vi "Convert RAWDATA.vi"(0 "Detector in":refnum<class "Detector.lvclass">, 1 "I channel":sgl[][](array[numeric]), 3 "WCM_values IN":sgl[](array[numeric]), 4 "II channel":sgl[][](array[numeric]), 5 "error in (no error)":errorcluster, 6 "# of scan":i32, 7 "All?":bool=TRUE, 10 "WCM_limits":T1, 11 "WCM_corrections":bool, 12 "I channel seq IN":cluster{"BG":sgl[], "Ie":sgl[], "I0":sgl[]}[](array[cluster]), 13 "II channel seq IN":cluster{"BG":sgl[], "Ie":sgl[], "I0":sgl[]}[](array[cluster])) -> (14 "Detector out":refnum<class "Detector.lvclass">, 15 "I channel seq":cluster{"BG":sgl[], "Ie":sgl[], "I0":sgl[]}[](array[cluster]), 17 "WCM_correction_coff":sgl[](array[numeric]), 18 "II channel seq":cluster{"BG":sgl[], "Ie":sgl[], "I0":sgl[]}[](array[cluster]), 19 "error out":errorcluster)   [LabVIEW 2020, in "Detector.lvclass"]
uses:
  Detector.lvclass
  dependecies/ControlsVIs/Clusters-def/Def_WCM_limits.ctl
  Detector.lvclass/Detector.ctl
  Read SC sum values ref.vi
  dependecies/globalVarII.vi
  <userlib>/_OpenG.lib/array/array.llb/Search 1D Array (SGL)__ogtk.vi
  Oscilloscope/Oscilloscope.lvclass
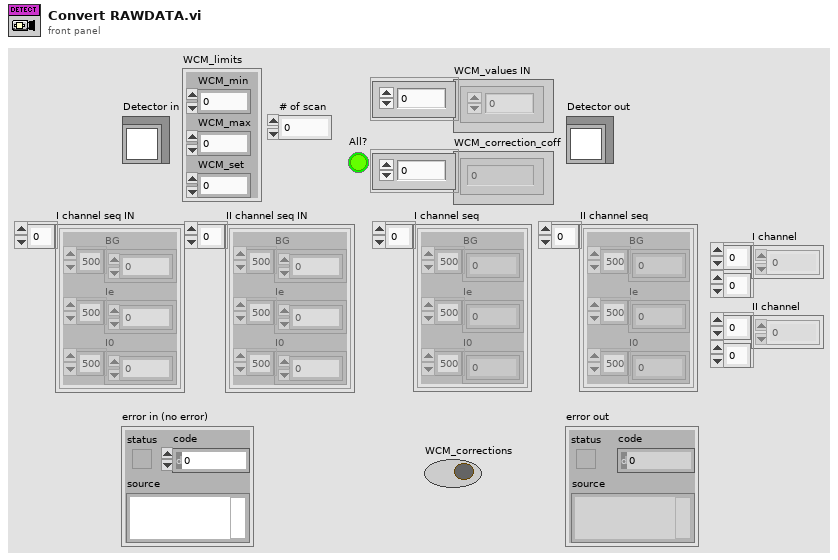
[diagram p1: front panel]
types:
  T1 = typedef "Oscilloscope.lvclass/Def_WCM_limits.ctl" = cluster{"WCM_min":dbl, "WCM_max":dbl, "WCM_set":dbl}
  T2 = typedef "Control-Client.lvclass/Controls-refs_CLIENT.ctl" = cluster{"ON/OFF Cool":refnum<vi>, "Save spectra":refnum<vi>, "Read detector":refnum<vi>, "# scans":refnum<vi>, "BG-level":refnum<vi>, "Set T":refnum<vi>, "Termometer":refnum<vi>, "Spectra":refnum<vi>, "Error Meter_ref":refnum<vi>, "OD graph":refnum<vi>, "from_pixel":refnum<vi>, "to_pixel":refnum<vi>, "threshold_ref_channel":refnum<vi>, "value":refnum<vi>, "python session":refnum<vi>, "ref h5_file":T3, "distance":refnum<vi>}
  T3 = typedef "hid_t.ctl" = i64
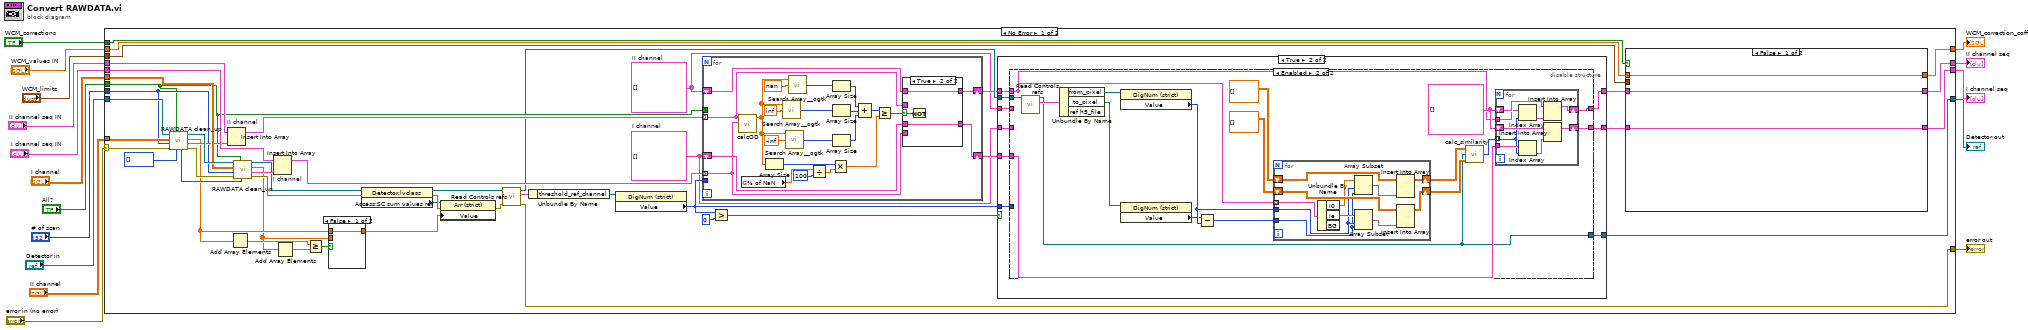
[diagram p0: block diagram]
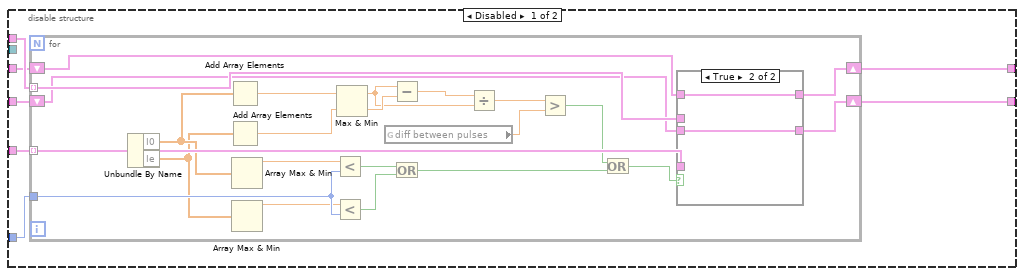
[diagram p3: hidden frame]
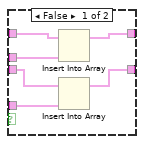
[diagram p4: hidden frame]
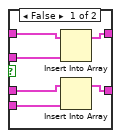
[diagram p5: hidden frame]
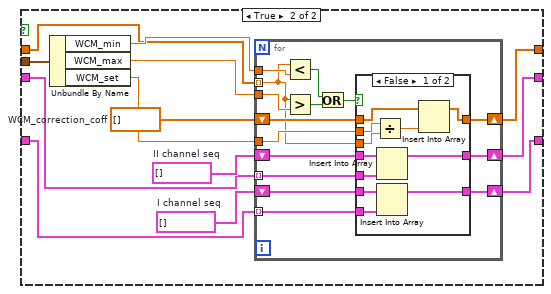
[diagram p7: hidden frame]
diagram:
  n1 = case shown="No Error" "error in (no error)" {
    selector: "error in (no error)" -> [w56 w235]
    tunnel: [w17 w236] -> w13
    tunnel: "Detector in" -> [w55 w236]
    tunnel: [w18 w235] -> w12
    tunnel: [w64 w234] -> w16
    tunnel: [w63 w233] -> w15
    tunnel: "II channel seq IN" -> [w62 w234]
    tunnel: "I channel seq IN" -> [w61 w233]
    tunnel: [w60 w232] -> w5
    tunnel: "WCM_values IN" -> [w59 w232]
    tunnel: "I channel" -> [w45 _]
    tunnel: "II channel" -> [w47 _]
    tunnel: "WCM_corrections" -> [w58 _]
    tunnel: "WCM_limits" -> [w57 _]
    tunnel: "All?" -> [w31 _]
    tunnel: "# of scan" -> [w38 _]
    frame No Error {
      w21 = cluster{"BG":sgl[], "Ie":sgl[], "I0":sgl[]}[] []  # II channel
      w22 = cluster{"BG":sgl[], "Ie":sgl[], "I0":sgl[]}[] []  # I channel
      n2 = call "RAWDATA clean_up.vi"("BG index IN"=i32[] [], "All?"=w31, "error in (no error)"=w56, "# of scan"=w38, "channel"=w47, "Detector in"=w55) -> ("error out"=w49:errorcluster, "channel seq"=w43:cluster{"BG":i32[], "Ie":i32[], "I0":i32[]}[], "SC values"=w39:sgl[], "Detector out"=w48:refnum<class "Detector.lvclass">, "BG indexes"=w46:i32[])  [unwired: 1 in]
      n3 = Insert Into Array "II channel"(array=w62, new element=w43) -> (w35:cluster{"BG":sgl[], "Ie":sgl[], "I0":sgl[]}[])  [unwired: 1 in]
      n4 = Add Array Elements(numeric array=w39) -> (sum=w52:sgl)
      n5 = call "RAWDATA clean_up.vi"("BG index IN"=w46, "All?"=w31, "error in (no error)"=w49, "# of scan"=w38, "channel"=w45, "Detector in"=w48) -> ("error out"=w41:errorcluster, "channel seq"=w44:cluster{"BG":i32[], "Ie":i32[], "I0":i32[]}[], "SC values"=w32:sgl[], "Detector out"=w42:refnum<class "Detector.lvclass">)  [unwired: 1 in, 1 out]
      n6 = Insert Into Array "I channel"(array=w61, new element=w44) -> (w36:cluster{"BG":sgl[], "Ie":sgl[], "I0":sgl[]}[])  [unwired: 1 in]
      n7 = Add Array Elements(numeric array=w32) -> (sum=w51:sgl)
      n8 = Greater Or Equal?(x=w52, y=w51) -> (x >= y?=w50:bool)
      n9 = case shown="False" w50 {
        tunnel: w39 -> [w185 _]
        tunnel: [w185 w186] -> w40
        tunnel: w32 -> [_ w186]
        frame False {
        }
        frame True {
        }
      }
      n10 = property class="Detector.lvclass"(reference=w42, error in=w41) -> (reference out=w29:refnum<class "Detector.lvclass">, error out=w54:errorcluster, "Access:SC sum values ref"=w53:refnum<vi>)
      n11 = property class="Arr (strict)"(reference=w53, error in=w54, "Value"=w40) -> (error out=w30:errorcluster)  [unwired: 1 out]
      n12 = call "Read Controls refs.vi"("error in (no error)"=w30, "Detector in"=w29) -> ("error out"=w18:errorcluster, "Controls refs"=w28:T2, "Detector out"=w25:refnum<class "Detector.lvclass">)  [unwired: 7 in]
      n13 = Unbundle By Name(w28) -> ("threshold_ref_channel"=w27:refnum<vi>)
      n14 = property class="DigNum (strict)"(reference=w27) -> ("Value"=w26:i32)  [unwired: 1 in, 2 out]
      n15 = for {
        tunnel: w36 -> [w155] mode=indexing
        tunnel: w35 -> [w165] mode=indexing
        shift-right: [w153] -> w23
        shift-left: w22 -> [w167]
        shift-right: [w154] -> w24
        shift-left: w21 -> [w166]
        tunnel: w31 -> [_]
        tunnel: w26 -> [_]
        n16 = call "calcOD.vi"("channel I"=w155, "channel 2"=w165) -> ("OD"=w173:sgl[])  [unwired: 3 in, 6 out]
        n17 = global read "globalVarII.vi" "% of NaN"() -> (w163:sgl)
        n18 = Array Size(array=w173) -> (size(s)=w172:i32)
        n19 = call-poly <userlib>:"Search Array__ogtk.vi"("Array"=w173, "Element Data"=sgl inf) -> ("Indices of Elements"=w171:i32[])  [unwired: 7 in]
        n20 = call-poly <userlib>:"Search Array__ogtk.vi"("Array"=w173, "Element Data"=sgl -inf) -> ("Indices of Elements"=w170:i32[])  [unwired: 7 in]
        n21 = call-poly <userlib>:"Search Array__ogtk.vi"("Array"=w173, "Element Data"=sgl nan) -> ("Indices of Elements"=w174:i32[])  [unwired: 7 in]
        n22 = Divide(x=w163, y=100) -> (x/y=w164:sgl)
        n23 = Multiply(x=w172, y=w164) -> (x*y=w157:sgl)
        n24 = Array Size(array=w174) -> (size(s)=w161:i32)
        n25 = Array Size(array=w171) -> (size(s)=w160:i32)
        n26 = Array Size(array=w170) -> (size(s)=w159:i32)
        n27 = Compound Arithmetic op=ADD(w161, w160, w159) -> (w158:i32)
        n28 = Greater Or Equal?(x=w158, y=w157) -> (x >= y?=w156:bool)
        n29 = case shown="True" w156 {
          selector: w156 -> [_ w182]
          tunnel: w167 -> [w181 w183]
          tunnel: w155 -> [w180 _]
          tunnel: [w179 w183] -> w153
          tunnel: [w178 w184] -> w154
          tunnel: w166 -> [w177 w184]
          tunnel: w165 -> [w176 _]
          frame False {
            n30 = Insert Into Array(array=w177, new element=w176) -> (w178:cluster{"BG":sgl[], "Ie":sgl[], "I0":sgl[]}[])  [unwired: 1 in]
            n31 = Insert Into Array(array=w181, new element=w180) -> (w179:cluster{"BG":sgl[], "Ie":sgl[], "I0":sgl[]}[])  [unwired: 1 in]
          }
          frame True {
            n32 = Not(x=w182) -> ()  [unwired: 1 out]
          }
        }
      }
      n33 = Greater?(x=w26, y=0) -> (0:w19:bool)
      n34 = case shown="True" w19 {
        tunnel: [w67 w72] -> w33
        tunnel: w24 -> [w67 w76]
        tunnel: w23 -> [w66 w75]
        tunnel: [w66 w71] -> w34
        tunnel: w22 -> [_ w74]
        tunnel: w21 -> [_ w73]
        tunnel: w26 -> [_ w70]
        tunnel: w25 -> [w65 w69]
        tunnel: [w65 w68] -> w17
        frame False {
        }
        frame True {
          n35 = disable-structure shown="Enabled" {
            disable-tunnel: w76 -> [w83 w126]
            disable-tunnel: w75 -> [w82 w129]
            disable-tunnel: w74 -> [w81 _]
            disable-tunnel: w73 -> [w80 _]
            disable-tunnel: [w79 w125] -> w72
            disable-tunnel: [w78 w128] -> w71
            disable-tunnel: w70 -> [w77 _]
            disable-tunnel: w69 -> [_ w121]
            disable-tunnel: [_ w115] -> w68
            frame Disabled {
              n36 = for {
                tunnel: w83 -> [w102] mode=indexing
                tunnel: w82 -> [w101] mode=indexing
                shift-right: [w99] -> w78
                shift-left: w81 -> [w100]
                shift-right: [w103] -> w79
                shift-left: w80 -> [w104]
                tunnel: w77 -> [w98]
                n37 = Unbundle By Name(w101) -> ("I0"=w93:sgl[], "Ie"=w92:sgl[])
                n38 = Add Array Elements(numeric array=w93) -> (sum=w91:sgl)
                n39 = Add Array Elements(numeric array=w92) -> (sum=w90:sgl)
                n40 = Array Max & Min(array=w93) -> (max value=w95:sgl)  [unwired: 3 out]
                n41 = Array Max & Min(array=w92) -> (max value=w94:sgl)  [unwired: 3 out]
                n42 = Less?(x=w95, y=w98) -> (x < y?=w105:bool)
                n43 = Less?(x=w94, y=w98) -> (x < y?=w106:bool)
                n44 = Max & Min(x=w91, y=w90) -> (max(x,y)=w87:sgl, min(x,y)=w89:sgl)
                n45 = global read "globalVarII.vi" "diff between pulses"() -> (w84:dbl)
                n46 = Subtract(x=w87, y=w89) -> (x-y=w88:sgl)
                n47 = Or(x=w105, y=w106) -> (x .or. y?=w97:bool)
                n48 = Divide(x=w88, y=w87) -> (x/y=w86:sgl)
                n49 = Greater?(x=w86, y=w84) -> (0:w85:bool)
                n50 = Or(x=w85, y=w97) -> (x .or. y?=w96:bool)
                n51 = case shown="True" w96 {
                  tunnel: w104 -> [w112 w114]
                  tunnel: [w111 w114] -> w103
                  tunnel: w102 -> [w110 _]
                  tunnel: w101 -> [w109 _]
                  tunnel: w100 -> [w108 w113]
                  tunnel: [w107 w113] -> w99
                  frame False {
                    n52 = Insert Into Array(array=w112, new element=w110) -> (w111:cluster{"BG":sgl[], "Ie":sgl[], "I0":sgl[]}[])  [unwired: 1 in]
                    n53 = Insert Into Array(array=w108, new element=w109) -> (w107:cluster{"BG":sgl[], "Ie":sgl[], "I0":sgl[]}[])  [unwired: 1 in]
                  }
                  frame True {
                  }
                }
              }
            }
            frame Enabled {
              w127 = cluster{"BG":sgl[], "Ie":sgl[], "I0":sgl[]}[] [] ("I channel")
              n54 = call "Read Controls refs.vi"("Detector in"=w121) -> ("Controls refs"=w120:T2, "Detector out"=w115:refnum<class "Detector.lvclass">)  [unwired: 8 in, 1 out]
              n55 = Unbundle By Name(w120) -> ("from_pixel"=w119:refnum<vi>, "to_pixel"=w118:refnum<vi>)  [unwired: 1 out]
              n56 = property class="DigNum (strict)"(reference=w119) -> ("Value"=w117:i32)  [unwired: 1 in, 2 out]
              n57 = property class="DigNum (strict)"(reference=w118) -> ("Value"=w116:i32)  [unwired: 1 in, 2 out]
              n58 = Subtract(x=w116, y=w117) -> (x-y=w122:i32)
              n59 = for {
                tunnel: w126 -> [w152] mode=indexing
                shift-right: [w150] -> w130
                shift-left: dbl[][] [] -> [w151]
                shift-right: [w148] -> w123
                shift-left: dbl[][] [] -> [w149]
                tunnel: w117 -> [w143]
                tunnel: w122 -> [w142]
                n60 = Unbundle By Name(w152) -> ("I0"=w145:sgl[], "Ie"=w147:sgl[])  [unwired: 1 out]
                n61 = Array Subset(array=w145, index=w143, length=w142) -> (w144:sgl[])
                n62 = Array Subset(array=w147, index=w143, length=w142) -> (w146:sgl[])
                n63 = Insert Into Array(array=w151, new element=w144) -> (w150:dbl[][])  [unwired: 2 in]
                n64 = Insert Into Array(array=w149, new element=w146) -> (w148:dbl[][])  [unwired: 2 in]
              }
              n65 = call "calc_similarity.vi"("data2"=w123, "Detector in"=w115, "data1"=w130) -> ("res out"=w124:i32[])
              n66 = for {
                tunnel: w129 -> [w141]
                shift-right: [w138] -> w128
                shift-left: w127 -> [w139]
                shift-right: [w137] -> w125
                shift-left: w127 -> [w136]
                tunnel: w126 -> [w135]
                tunnel: w124 -> [w133] mode=indexing
                n67 = Index Array(array=w135, index=w133) -> (element=w134:cluster{"BG":sgl[], "Ie":sgl[], "I0":sgl[]})
                n68 = Index Array(array=w141, index=w133) -> (element=w140:cluster{"BG":sgl[], "Ie":sgl[], "I0":sgl[]})
                n69 = Insert Into Array(array=w136, new element=w134) -> (w137:cluster{"BG":sgl[], "Ie":sgl[], "I0":sgl[]}[])  [unwired: 1 in]
                n70 = Insert Into Array(array=w139, new element=w140) -> (w138:cluster{"BG":sgl[], "Ie":sgl[], "I0":sgl[]}[])  [unwired: 1 in]
              }
            }
          }
        }
      }
      n71 = case shown="False" w58 {
        tunnel: [w189 w194] -> w64
        tunnel: w33 -> [w189 w196]
        tunnel: [w188 w195] -> w63
        tunnel: w34 -> [w188 w197]
        tunnel: [w187 w193] -> w60
        tunnel: w59 -> [w187 w192]
        tunnel: w57 -> [_ w191]
        frame False {
        }
        frame True {
          w201 = cluster{"BG":i32[], "Ie":i32[], "I0":i32[]}[] []  # II channel seq
          w202 = cluster{"BG":i32[], "Ie":i32[], "I0":i32[]}[] []  # I channel seq
          w198 = sgl[] []  # WCM_correction_coff
          n72 = Unbundle By Name(w191) -> ("WCM_min"=w200:dbl, "WCM_max"=w199:dbl, "WCM_set"=w190:dbl)
          n73 = for {
            tunnel: w199 -> [w216]
            tunnel: w200 -> [w217]
            shift-right: [w214] -> w193
            shift-left: w198 -> [w215]
            shift-right: [w208] -> w194
            shift-left: w201 -> [w207]
            shift-right: [w209] -> w195
            shift-left: w202 -> [w210]
            tunnel: w197 -> [w206] mode=indexing
            tunnel: w196 -> [w205] mode=indexing
            tunnel: w192 -> [w203] mode=indexing
            tunnel: w190 -> [w204]
            n74 = Less?(x=w203, y=w217) -> (x < y?=w213:bool)
            n75 = Greater?(x=w203, y=w216) -> (0:w212:bool)
            n76 = Or(x=w213, y=w212) -> (x .or. y?=w211:bool)
            n77 = case shown="False" w211 {
              tunnel: [w227 w231] -> w214
              tunnel: w215 -> [w228 w231]
              tunnel: w210 -> [w226 w230]
              tunnel: [w225 w230] -> w209
              tunnel: [w223 w229] -> w208
              tunnel: w207 -> [w224 w229]
              tunnel: w206 -> [w222 _]
              tunnel: w205 -> [w221 _]
              tunnel: w204 -> [w220 _]
              tunnel: w203 -> [w219 _]
              frame False {
                n78 = Divide(x=w220, y=w219) -> (x/y=w218:dbl)
                n79 = Insert Into Array(array=w224, new element=w221) -> (w223:cluster{"BG":i32[], "Ie":i32[], "I0":i32[]}[])  [unwired: 1 in]
                n80 = Insert Into Array(array=w226, new element=w222) -> (w225:cluster{"BG":i32[], "Ie":i32[], "I0":i32[]}[])  [unwired: 1 in]
                n81 = Insert Into Array(array=w228, new element=w218) -> (w227:sgl[])  [unwired: 1 in]
              }
              frame True {
              }
            }
          }
        }
      }
    }
    frame Error {
    }
  }
  "error out" <- w12
  "Detector out" <- w13
  "WCM_correction_coff" <- w5
  "II channel seq" <- w16
  "I channel seq" <- w15
